vi "crio_RT_VCA_Closed_Loop_Vibration_Injection.vi"() -> ()   [LabVIEW 2019]
uses:
  <vilib>/LabVIEW Targets/FPGA/cRIO/shared/nicrio_ModuleControls/nicrio_cRIO-9237_ExcitationVoltageRing.ctl
  <vilib>/Platform/TimedLoop/XDataNode/timing_clust.ctl
  <vilib>/Platform/TimedLoop/XDataNode/nitl_modes.ctl
  <vilib>/Platform/TimedLoop/XDataNode/wakeup.ctl
  <vilib>/FPGAPlugInAG/cRIO-9074/niLvFpga_Open_cRIO-9074.vi
  <vilib>/rvi/interface/common/dynamic/niFpgaDynamicAddResources.vi
  <vilib>/Utility/error.llb/Error Cluster From Error Code.vi
  <vilib>/rvi/errors/niLvFpgaAdjustHostInterfaceError.vi
  <vilib>/FPGAPlugInAG/Dynamic/niLvFpga_Close_Dynamic.vi
  <vilib>/rvi/interface/nirviOpenFPGA/nirviOpenFPGA.xnode
  On Call Bitfiles/gpass2_FPGATarget2_crioFPGAAntagoni_uWzRZvtrb5U.lvbitx
  <vilib>/rvi/interface/nirviReadWriteControl/nirviReadWriteControl.xnode
  <vilib>/platform/TimedLoop/XDataNode/XDataNode.xnode
  <vilib>/rvi/interface/nirviCloseFPGA/nirviCloseFPGA.xnode
  NiFpgaLv.dll
  <vilib>/rvi/interface/Simulation/niFpgaSimulationCallBeginRW.vi
  <vilib>/Platform/TimedLoop/XDataNode/XDNodeRunTimeDep.lvlib
panel:
  in  "Default sin gain":dbl=20.0
  out "rail Platform Position":i16=4000
  out "LAC Measured Position":i32
  in  "VCA Loop Period(us)":i64=2000
  in  "VCA Position Reset":bool
  in  "VCA Velocity Interval (uSec)":u32=1000
  in  "LAC Position Reset":bool
  in  "LAC Velocity Interval (uSec)":u32=1000
  in  "LAC Lock":bool
  in  "Rail Manual Operation":bool
  in  "Rail Stepper Enable":bool
  in  "Rail Stepper Direction":bool
  in  "Half Peirod (pulse 40MHz)":u32=10000
  out "LAC Actual Gain":T1={"proportional gain"=0.009545455, "integral gain"=1.2626262e-09}
  in  "LAC manual control":T2={"manual? (F)"=FALSE, "manual input (0)"=-0.83838385} {"manual input (0)" scale=-1.0..1.0}
  in  "LAC setpoint":i32(slide)=2700 scale=0.0..4500.0
  in  "LAC Gains":T1={"proportional gain"=0.95454544, "integral gain"=0.64646465} {"proportional gain" scale=0.0..1.0; "integral gain" scale=0.0..1.0}
  in  "LAC Gain Scaler":T1={"proportional gain"=100.0, "integral gain"=100000000.0}
  in  "Rail Desired Position":i16(slide)=4000 scale=0.0..20000.0
  in  "PWM Frequency (default 20kHz)":i32=20000
  in  "Excitation Voltage":T3 items=["2.5 Volts", "3.3 Volts", "5.0 Volts", "10.0 Volts", "External Excitation"]
  out "scaled load cell reading":fxp<+/-,24,24>
  in  "VCA Manual Control":T2
  in  "VCA Gains":T1={"proportional gain"=0.25, "integral gain"=0.7979798} {"proportional gain" scale=0.0..1.0; "integral gain" scale=0.0..1.0}
  out "VCA Actual Gain":T1={"proportional gain"=0.0009797979, "integral gain"=7.979798e-09}
  in  "VCA Gain Scaler":T1={"proportional gain"=1000.0, "integral gain"=100000000.0}
  out "VCA Force Setpoint":sgl
  out "VCA Force":dbl(graph)
  out "PWM":sgl(graph)=0.061072454
  out "ControllerPWM Output":sgl=0.061072454
  out "ms to next point":u32=50500
  in  "Start Fequency":dbl=0.2
  out "Current Sweeping frequency":dbl=0.2
  in  "End Frequency":i32=20
  in  "Frequency Increment":dbl=1.0
  in  "Start Sweep":bool
  in  "Frequency":dbl=0.2
  in  "Lock_loop_rate":u32=5000
  in  "sin_gain":fxp<+,32,10>=0.25
  in  "sin_offset":fxp<+/-,32,10>=0.5
  in  "stop":bool
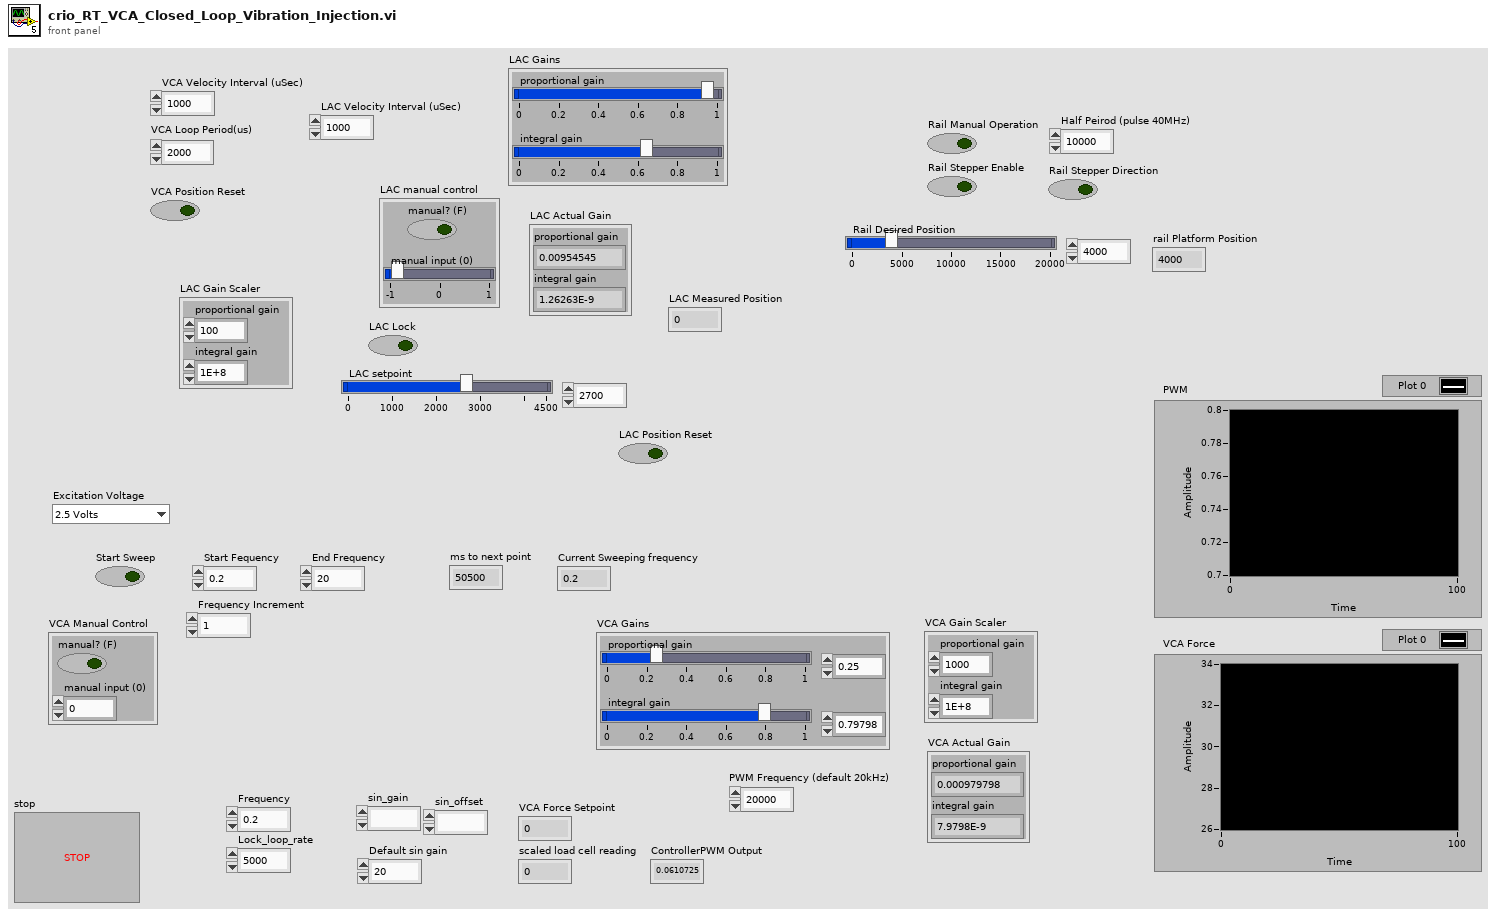
[diagram p1: front panel]
types:
  T1 = cluster{"proportional gain":sgl, "integral gain":sgl}
  T2 = cluster{"manual? (F)":bool, "manual input (0)":sgl}
  T3 = typedef "nicrio_cRIO-9237_ExcitationVoltageRing.ctl" = u8
  T4 = typedef "XDNodeRunTimeDep.lvlib/timing_clust.ctl" = cluster{"Expected End [f-1]":u64, "Actual End [f-1]":u64, "Finished Late? [f-1]":bool, "Expected End [i-1]":u64, "Actual End [i-1]":u64, "Finished Late? [i-1]":bool, "Expected Start [i]":u64, "Actual Start [i]":u64, "Expected Start [f]":u64, "Actual Start [f]":u64, "Source Name":string, "Structure Name":string, "Period":i64, "Deadline":i64, "Offset":i64, "Start":i64, "Priority":i32, "Timeout":i32, "Mode":T5, "Wakeup Reason":T6, "Error":errorcluster, "Source Type":string, "Secondary Source Type":string, "Global End Time":u64, "Global Start Time":u64, "Frame Duration":u64, "Iteration Duration":u64, "Assigned CPU":i32, "I/O Scan Engine Mode":u32}
  T5 = typedef "XDNodeRunTimeDep.lvlib/nitl_modes.ctl" = enum32{"No Change", "Process missed periods, maintain original phase", "Discard missed periods, maintain original phase", "Process missed periods, ignore original phase", "Discard missed periods, ignore original phase"}
  T6 = typedef "XDNodeRunTimeDep.lvlib/wakeup.ctl" = enum32{"Normal", "Aborted", "Asynchronous wakeup", "Timing source error", "Timed loop error", "Timeout"}
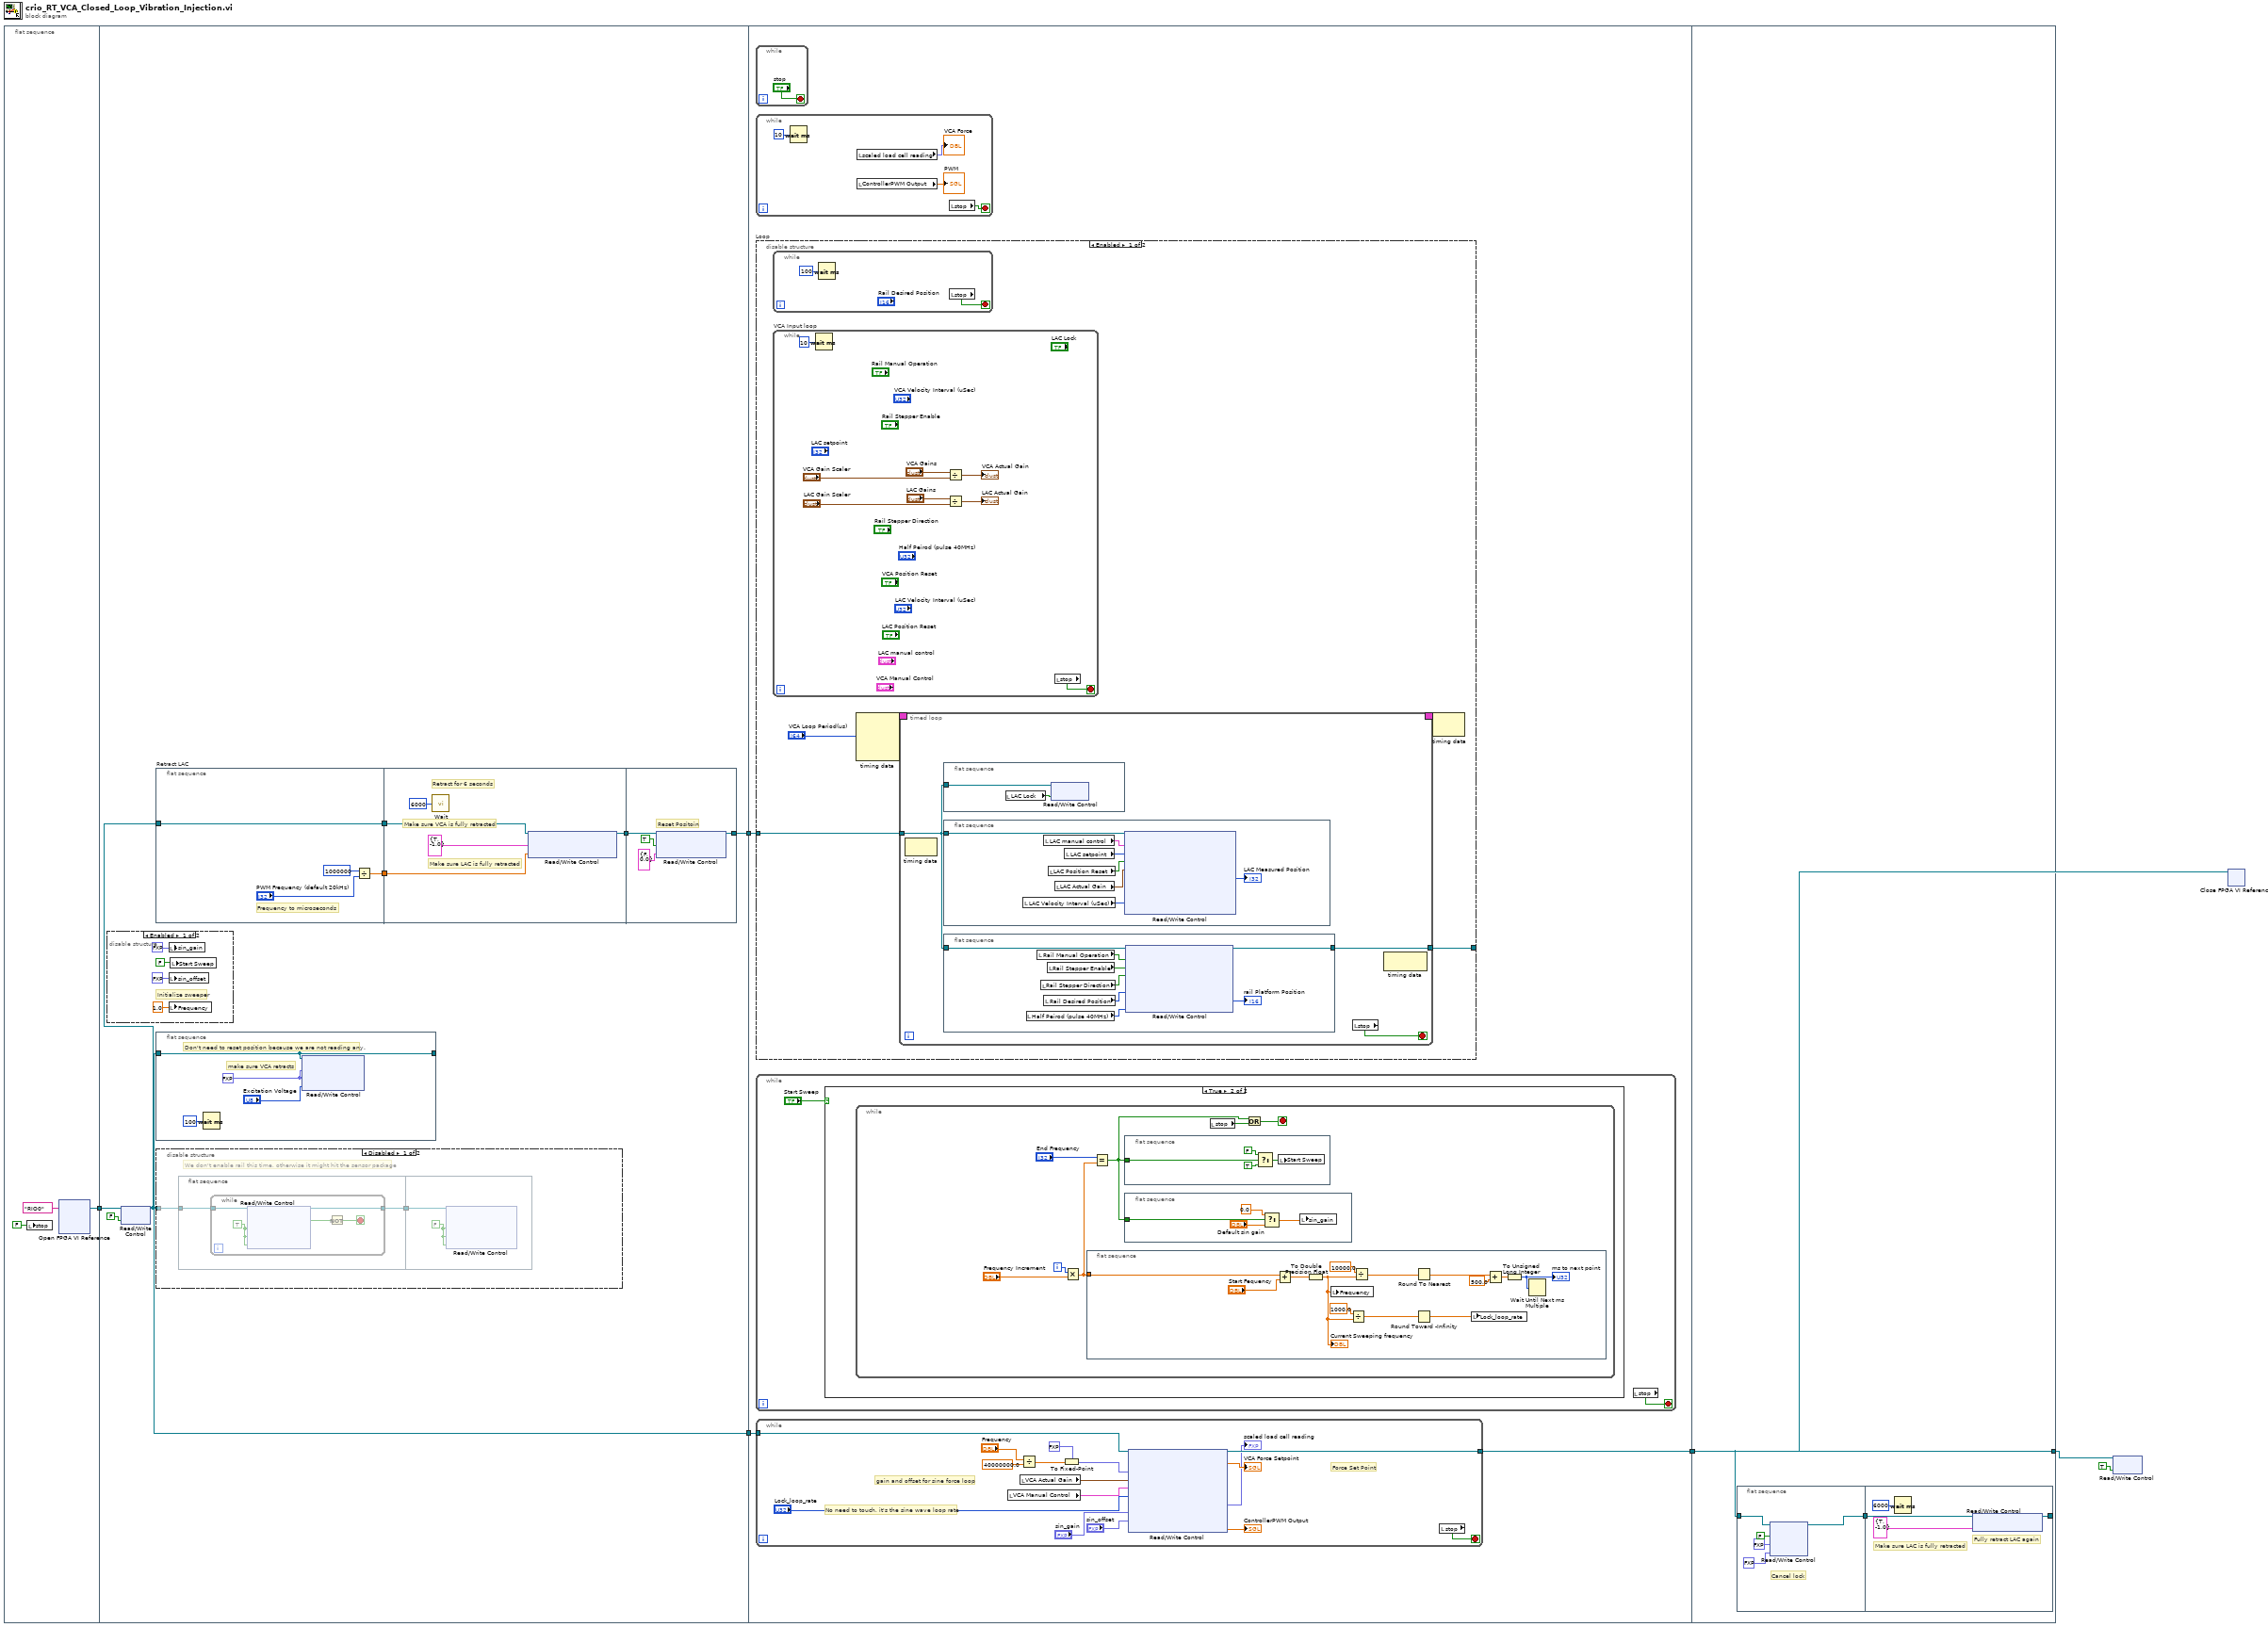
[diagram p0: block diagram]
diagram:
  n1 = flat-sequence {
    tunnel: [w9] -> w6
    tunnel: w6 -> [w15]
    tunnel: [w11] -> w5
    tunnel: [w10] -> w3
    tunnel: w5 -> [w51]
    tunnel: [w50] -> w4
    tunnel: w3 -> [w49]
    tunnel: w4 -> [w144]
    tunnel: [w144] -> w1
    frame #0 {
      n2 = local write "stop"(FALSE ("stop")) -> ()
      n3 = xnode "Open FPGA VI Reference"("resource name"=tag "RIO0") -> ("FPGA VI Reference Out"=w9:refnum<k20>)  [unwired: 1 in, 1 out]
    }
    frame #1 {
      n4 = disable-structure shown="Enabled" {
        frame Enabled {
          # "Initialize sweeper"
          n5 = local write "sin_gain"(fxp<+,16,2> 0.0 ("sin_gain")) -> ()
          n6 = local write "sin_offset"(fxp<+/-,16,3> 0.0 ("sin_offset")) -> ()
          n7 = local write "Frequency"(1.0 ("Frequency")) -> ()
          n8 = local write "Start Sweep"(FALSE ("Start Sweep")) -> ()
        }
        frame Disabled {
        }
      }
      n9 = xnode "Read/Write Control"("FPGA VI Reference In"=w15, "stop"=FALSE) -> ("FPGA VI Reference Out"=w11:refnum<k20>)  [unwired: 1 in, 1 out]
      n10 = flat-sequence "Retract LAC" {
        tunnel: [w23] -> w14
        tunnel: w11 -> [w21]
        tunnel: [w21] -> w13
        tunnel: w14 -> [w28]
        tunnel: w13 -> [w26]
        tunnel: [w29] -> w12
        tunnel: w12 -> [w32]
        tunnel: [w33] -> w10
        frame #0 {
          # "Frequency to microseconds"
          n11 = Divide(x=1000000, y="PWM Frequency (default 20kHz)") -> (x/y=w23:dbl)
        }
        frame #1 {
          # "Make sure LAC is fully retracted"
          # "Retract for 6 seconds"
          # "Make sure VCA is fully retracted"
          n12 = call "Wait"("Count(mSec)"=u32 6000) -> ()  [unwired: 1 out]
          n13 = xnode "Read/Write Control"("FPGA VI Reference In"=w26, "LAC Manual Control"=T2 {"manual? (F)"=TRUE, "manual input (0)"=-1.0} ("manual control"), "DC PWM Period (microsec)"=w28) -> ("FPGA VI Reference Out"=w29:refnum<k20>)  [unwired: 1 in, 1 out]
        }
        frame #2 {
          # "Reset Positoin"
          n14 = xnode "Read/Write Control"("FPGA VI Reference In"=w32, "Position Reset"=TRUE, "LAC Manual Control"=T2 {"manual? (F)"=FALSE, "manual input (0)"=0.0} ("manual control")) -> ("FPGA VI Reference Out"=w33:refnum<k20>)  [unwired: 1 in, 1 out]
        }
      }
      n15 = flat-sequence {
        tunnel: [w45] -> _
        tunnel: w11 -> [w45]
        frame #0 {
          w48 = fxp<+/-,16,3> 0.0 ("sin_offset")
          # "Don't need to reset position because we are not reading any."
          # "make sure VCA retracts"
          n16 = Wait (ms)(milliseconds to wait=u32 100) -> ()  [unwired: 1 out]
          n17 = xnode "Read/Write Control"("FPGA VI Reference In"=w45, "sin_offset"=w48, "sin_gain"=w48, "Excitation Voltage"="Excitation Voltage") -> ()  [unwired: 1 in, 2 out]
        }
      }
      n18 = disable-structure shown="Disabled" {
        disable-tunnel: w11 -> [w34 _]
        frame Disabled {
          # "We don't enable rail this time, otherwise it might hit the sensor package"
          n19 = flat-sequence {
            tunnel: w34 -> [w36]
            tunnel: [w37] -> w35
            tunnel: w35 -> [w44]
            frame #0 {
              n20 = while {
                tunnel: [w41] -> w37
                tunnel: w36 -> [w40]
                stop <- w38 stop-if-true
                w42 = TRUE ("Stepper Direction")
                n21 = xnode "Read/Write Control"("FPGA VI Reference In"=w40, "Manual Operation"=w42, "Stepper Enable"=w42, "Stepper Direction"=w42) -> ("FPGA VI Reference Out"=w41:refnum<k20>, "Limit Switch"=w39:bool)  [unwired: 1 in, 1 out]
                n22 = Not(x=w39) -> (.not. x?=w38:bool)
              }
            }
            frame #1 {
              w43 = FALSE ("Stepper Direction")
              n23 = xnode "Read/Write Control"("FPGA VI Reference In"=w44, "Manual Operation"=w43, "Stepper Enable"=w43, "Stepper Direction"=w43) -> ()  [unwired: 1 in, 3 out]
            }
          }
        }
        frame Enabled {
          # "We don't enable rail this time, otherwise it might hit the sensor package"
        }
      }
    }
    frame #2 {
      n24 = while {
        stop <- "stop" stop-if-true
      }
      n25 = while {
        stop <- w95 stop-if-true
        n26 = Wait (ms)(milliseconds to wait=u32 10) -> ()  [unwired: 1 out]
        n27 = local read "scaled load cell reading"() -> (→"VCA Force":fxp<+/-,24,24>)
        n28 = local read "ControllerPWM Output"() -> (→"PWM":sgl)
        n29 = local read "stop"() -> (w95:bool)
      }
      n30 = disable-structure "Loop" shown="Enabled" {
        disable-tunnel: w49 -> [w53 _]
        disable-tunnel: [w52 _] -> _
        frame Enabled {
          n31 = while {
            stop <- w57 stop-if-true
            n32 = Wait (ms)(milliseconds to wait=u32 100) -> ()  [unwired: 1 out]
            n33 = local read "stop"() -> (w57:bool)
          }
          n34 = while "VCA Input loop" {
            stop <- w65 stop-if-true
            n35 = Wait (ms)(milliseconds to wait=u32 10) -> ()  [unwired: 1 out]
            n36 = Divide(x="VCA Gains", y="VCA Gain Scaler") -> (x/y=→"VCA Actual Gain":T1)
            n37 = Divide(x="LAC Gains", y="LAC Gain Scaler") -> (x/y=→"LAC Actual Gain":T1)
            n38 = local read "stop"() -> (w65:bool)
          }
          n39 = node-c288("VCA Loop Period(us)") -> (w56:T4)  [unwired: 3 in]
          n40 = timed-loop {
            timing: w56 -> [_]
            timing-out: [_] -> w55
            tunnel: w53 -> [w67]
            tunnel: [w68] -> w52
            stop <- w69 stop-if-true
            n41 = node-c288() -> ()  [unwired: 1 in, 1 out]
            n42 = flat-sequence {
              tunnel: w67 -> [w86]
              frame #0 {
                n43 = local read "LAC Lock"() -> (w85:bool)
                n44 = xnode "Read/Write Control"("FPGA VI Reference In"=w86, "LAC Lock"=w85) -> ()  [unwired: 1 in, 2 out]
              }
            }
            n45 = flat-sequence {
              tunnel: w67 -> [w76]
              frame #0 {
                n46 = local read "LAC Velocity Interval (uSec)"() -> (w71:u32)
                n47 = local read "LAC manual control"() -> (w75:T2)
                n48 = local read "LAC Position Reset"() -> (w73:bool)
                n49 = local read "LAC Actual Gain"() -> (w72:T1)
                n50 = local read "LAC setpoint"() -> (w74:i32)
                n51 = xnode "Read/Write Control"("FPGA VI Reference In"=w76, "LAC Manual Control"=w75, "LAC Setpoint"=w74, "Position Reset"=w73, "LAC Gains"=w72, "LAC Velocity Interval (uSec)"=w71) -> ("LAC Position (Counts)"=→"LAC Measured Position":i32)  [unwired: 1 in, 5 out]
              }
            }
            n52 = flat-sequence {
              tunnel: w67 -> [w78]
              tunnel: [w77] -> w68
              frame #0 {
                n53 = local read "Half Peirod (pulse 40MHz)"() -> (w84:u32)
                n54 = local read "Rail Manual Operation"() -> (w80:bool)
                n55 = local read "Rail Stepper Direction"() -> (w81:bool)
                n56 = local read "Rail Desired Position"() -> (w83:i16)
                n57 = local read "Rail Stepper Enable"() -> (w82:bool)
                n58 = xnode "Read/Write Control"("FPGA VI Reference In"=w78, "Manual Operation"=w80, "Stepper Enable"=w82, "Stepper Direction"=w81, "Position Control: Desired Positoin"=w83, "Half Peirod (pulse 40MHz)"=w84) -> ("FPGA VI Reference Out"=w77:refnum<k20>, "rail Platform Position"=→"rail Platform Position":i16)  [unwired: 2 in, 1 out]
              }
            }
            n59 = local read "stop"() -> (w69:bool)
            n60 = node-c288() -> ()  [unwired: 1 in, 1 out]
          }
          n61 = node-c288(w55) -> ()  [unwired: 1 out]
        }
        frame Disabled {
        }
      }
      n62 = while {
        stop <- w98 stop-if-true
        n63 = case shown="True" "Start Sweep" {
          frame False {
          }
          frame True {
            n64 = while {
              i -> [w102]
              stop <- w105 stop-if-true
              n65 = Multiply(x=w102, y="Frequency Increment") -> (x*y=w101:dbl)
              n66 = flat-sequence {
                tunnel: w101 -> [w119]
                frame #0 {
                  n67 = Add(x=w119, y="Start Fequency") -> (x+y=w120:dbl)
                  n68 = To Double Precision Float(number=w120) -> (double precision float=w114:dbl)
                  "Current Sweeping frequency" <- w114
                  n69 = local write "Frequency"(w114) -> ()
                  n70 = Divide(x=1000.0 ("y"), y=w114) -> (x/y=w117:dbl)
                  n71 = Divide(x=10000.0 ("y"), y=w114) -> (x/y=w126:dbl)
                  n72 = Round To Nearest(number=w126) -> (nearest integer value=w123:dbl)
                  n73 = Round Toward -Infinity(1:w117) -> (0:w116:dbl)
                  n74 = local write "Lock_loop_rate"(w116) -> ()
                  n75 = Add(x=w123, y=500.0) -> (x+y=w121:dbl)
                  n76 = To Unsigned Long Integer(number=w121) -> (unsigned 32bit integer=w124:u32)
                  "ms to next point" <- w124
                  n77 = Wait Until Next ms Multiple(millisecond multiple=w124) -> ()  [unwired: 1 out]
                }
              }
              n78 = Equal?(x="End Frequency", y=w101) -> (x = y?=w99:bool)
              n79 = flat-sequence {
                tunnel: w99 -> [w113]
                frame #0 {
                  n80 = Select(t=FALSE, s=w113, f=TRUE) -> (s? t:f=w111:bool)
                  n81 = local write "Start Sweep"(w111) -> ()
                }
              }
              n82 = flat-sequence {
                tunnel: w99 -> [w109]
                frame #0 {
                  n83 = Select(t=0.0, s=w109, f="Default sin gain") -> (s? t:f=w108:dbl)
                  n84 = local write "sin_gain"(w108) -> ()
                }
              }
              n85 = local read "stop"() -> (w104:bool)
              n86 = Or(x=w99, y=w104) -> (x .or. y?=w105:bool)
            }
          }
        }
        n87 = local read "stop"() -> (w98:bool)
      }
      n88 = while {
        tunnel: w51 -> [w141]
        tunnel: [w132] -> w50
        stop <- w142 stop-if-true
        # "Force Set Point"
        # "gain and offset for sine force loop"
        # "No need to touch, it's the sine wave loop rate"
        n89 = local read "VCA Manual Control"() -> (w128:T2)
        n90 = local read "VCA Actual Gain"() -> (w129:T1)
        n91 = Divide(x="Frequency", y=40000000.0) -> (x/y=w139:dbl)
        n92 = To Fixed-Point(fixed-point type=fxp<+,32,0> 0.0 ("frequency (periods/tick)"), number=w139) -> (fixed-point=w136:fxp<+,32,0>)
        n93 = xnode "Read/Write Control"("FPGA VI Reference In"=w141, "sweep frequency (periods/tick)"=w136, "VCA Gains"=w129, "VCA Manual Control"=w128, "Lock_loop_rate"="Lock_loop_rate", "sin_gain"="sin_gain", "sin_offset"="sin_offset") -> ("FPGA VI Reference Out"=w132:refnum<k20>, "VCA Force Setpoint"=→"VCA Force Setpoint":sgl, "scaled load cell reading"=→"scaled load cell reading":fxp<+/-,24,24>, "VCA ControllerPWM Output"=→"ControllerPWM Output":sgl)  [unwired: 1 in, 1 out]
        n94 = local read "stop"() -> (w142:bool)
      }
    }
    frame #3 {
      n95 = flat-sequence {
        tunnel: w144 -> [w150]
        tunnel: [w149] -> w145
        tunnel: [w153] -> _
        tunnel: w145 -> [w154]
        frame #0 {
          # "Cancel lock"
          n96 = xnode "Read/Write Control"("FPGA VI Reference In"=w150, "LAC Lock"=FALSE, "sin_offset"=fxp<+/-,16,3> -1.0, "sin_gain"=fxp<+,32,1> 0.0) -> ("FPGA VI Reference Out"=w149:refnum<k20>)  [unwired: 1 in, 1 out]
        }
        frame #1 {
          # "Make sure LAC is fully retracted"
          # "Fully retract LAC again"
          n97 = Wait (ms)(milliseconds to wait=u32 6000) -> ()  [unwired: 1 out]
          n98 = xnode "Read/Write Control"("FPGA VI Reference In"=w154, "LAC Manual Control"=T2 {"manual? (F)"=TRUE, "manual input (0)"=-1.0} ("manual control")) -> ("FPGA VI Reference Out"=w153:refnum<k20>)  [unwired: 1 in, 1 out]
        }
      }
    }
  }
  n99 = xnode "Read/Write Control"("FPGA VI Reference In"=w1, "stop"=TRUE) -> ()  [unwired: 1 in, 2 out]
  n100 = xnode "Close FPGA VI Reference"("FPGA VI Reference In"=w1) -> ()  [unwired: 1 in, 1 out]
